vi "Fct_Limite_Pluie.vi"(11 "Pluie":dbl) -> (2 "Booléen":bool, 3 "Chaîne":string)   [LabVIEW 2017]
doc: "Ce VI gère les alarmes lié à la pluviométrie (Limites + Raisons des alarmes)\n\nCopyright | Jixiong Liu & Benoit Mangeard"
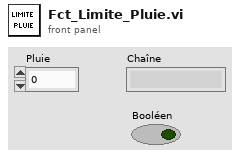
[diagram p1: front panel]
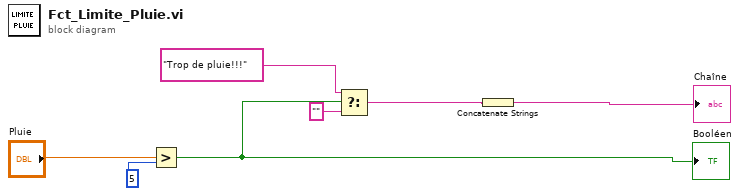
[diagram p0: block diagram]
diagram:
  n1 = Greater?(x="Pluie", y=5) -> (0:w1:bool)
  "Booléen" <- w1
  n2 = Select(t="Trop de pluie!!!", s=w1, f="" ("cas faux")) -> (s? t:f=w6:string)
  n3 = Concatenate Strings(w6) -> (→"Chaîne":string)
